vi "Memory.Array.Bounds Check.Length.vi"(8 "error in (no error)":errorcluster, 10 "length":i64=-1 format="%d bytes", 11 "Array in":refnum<class "Memory.Array.lvclass">) -> (0 "error out":errorcluster, 1 "length valid":bool, 2 "length out":i64=-1 format="%d bytes", 3 "Array out":refnum<class "Memory.Array.lvclass">)   [LabVIEW 2016, in "LabVIEW Memory Manager.lvlib" / "Memory.Array.lvclass"]
uses:
  Memory.Array.lvclass
  Memory.Array.lvclass/Memory.Array.ctl
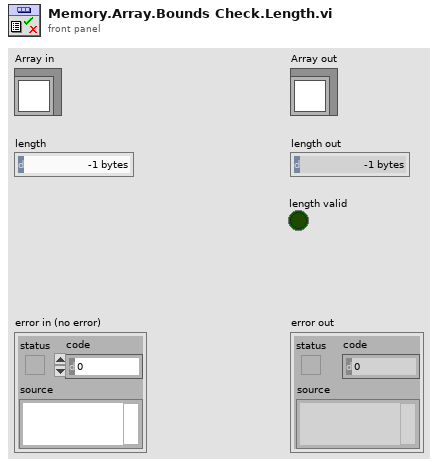
[diagram p1: front panel]
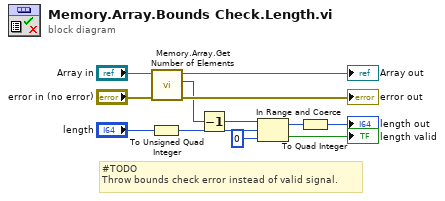
[diagram p0: block diagram]
diagram:
  # "#TODO\nThrow bounds check error instead of valid signal."
  n1 = To Unsigned Quad Integer(1:"length") -> (0:w3:u64)
  n2 = call "Memory.Array.Get Number of Elements.vi"("error in (no error)"="error in (no error)", "Memory.Array in"="Array in") -> ("error out"=→"error out":errorcluster, "number of elements"=w6:u64, "Memory.Array out"=→"Array out":refnum<class "Memory.Array.lvclass">)  [unwired: 7 in]
  n3 = Decrement(x=w6) -> (x-1=w11:u64)
  n4 = In Range and Coerce(upper limit=w11, x=w3, lower limit=u64 0) -> (coerced(x)=w5:u64, In Range?=→"length valid":bool)
  n5 = To Quad Integer(1:w5) -> (0:→"length out":i64)
